vi "filteredWhiteNoise.vi"(9 "frequency":dbl=0.5, 10 "offset":dbl, 11 "amplitude":dbl) -> (2 "Noise":dbl, 3 "Binary Noise":dbl)   [LabVIEW 2020]
uses:
  <vilib>/Simulation/Implementation/Shared/SIMSCR Execution Mode.ctl
  <vilib>/Simulation/Scripting/Companion Diagram/SimConfigNode/SimParams.ctl
  <vilib>/Simulation/Scripting/Companion Diagram/SimConfigNode/_simSolvers.ctl
  <vilib>/Simulation/Param Hierarchy/Typedefs/SIMPH Param Control Actions.ctl
  <vilib>/Simulation/Implementation/Shared/NILVSim_ParamChanged.vi
  <vilib>/Simulation/Implementation/Shared/NILVSim_FinishedLate.vi
  <vilib>/Simulation/Implementation/Shared/NILVSIM_BeginStep.vi
  <vilib>/Simulation/DataSources/Implementation/NILVSim Signal Generator.llb/SIM Signal Generator (scalar).vi
  <vilib>/Simulation/ContinuousLinear/Implementation/NILVSim Transfer Function.llb/SIM Transfer Function Distributor (SISO CD).vi
  <vilib>/Simulation/ContinuousLinear/Implementation/NILVSim Transfer Function.llb/SIM Transfer Function Collector (SISO).vi
  <vilib>/Simulation/Implementation/Shared/SIM Is Init or Final Stage.vi
  <vilib>/Simulation/SignalDisplay/Implementation/NILVSim Time Waveform.llb/SIM Time Waveform (vector).vi
  <vilib>/Simulation/Implementation/Shared/NILVSim_Manager.vi
  <vilib>/Utility/error.llb/Clear Errors.vi
  <vilib>/Simulation/Implementation/Shared/NILVSim_FinalizeModel.vi
  <vilib>/Simulation/Implementation/Shared/SIM Unbundle Sim Info.vi
  <vilib>/Simulation/Implementation/Shared/NILVSim_Initialize.vi
  <vilib>/addons/Control Design/_Model Construction/Special Model Creation.llb/Special Model Creation SubVI/CD Create 1st Order Model.vi
  <vilib>/addons/Control Design/_Frequency Response Analysis/Frequency Response.llb/Frequency Response subVI/cd_Bode (Transfer Function).vi
  <vilib>/addons/Control Design/_Frequency Response Analysis/Frequency Response.llb/Frequency Response subVI/cd_Bandwidth (Transfer Function).vi
  <vilib>/Simulation/Utility/Implementation/NILVSim Get Time and IsAcceptedStep.vi
  <vilib>/Simulation/Implementation/Shared/NILVSim_GetModelError.vi
  <vilib>/Simulation/Implementation/Shared/SIM SimErrorHandler.vi
  <vilib>/Simulation/Implementation/Shared/SIMSH Read Queue.vi
  <vilib>/Simulation/Implementation/Shared/SIM Bundle Sim Info.vi
  <vilib>/Simulation/Scripting/Companion Diagram/SimConfigNode/SimDog.xnode
  <vilib>/Simulation/Implementation/XNodeFramework/SimXNode/SimX.xnode
  <vilib>/addons/Control Design/_Model Construction/NI_CD_Special Model Creation.lvlib
  <vilib>/addons/Control Design/_Model Construction/Model Typedefs.llb/CD General Elements.ctl
  <vilib>/addons/Control Design/_Model Construction/NI_LinSys_Model Typedefs.lvlib
  <vilib>/addons/Control Design/_Model Construction/Model Typedefs.llb/CD Transfer Function Model (SISO).ctl
  <vilib>/addons/Control Design/_Model Construction/Model Typedefs.llb/CD Transfer Function Model (MIMO).ctl
  <vilib>/addons/Control Design/_Frequency Response Analysis/NI_CD_Frequency Response.lvlib
  <vilib>/Simulation/ContinuousLinear/Implementation/NILVSim Transfer Function.llb/SIM Transfer Function (SISO CD).vi
  <vilib>/Simulation/Implementation/Shared/NI_SIM_Implementation.lvlib
panel:
  out "rad/s":dbl
  out "Bode Magnitude":cluster{"W":dbl[], "Magnitude":dbl[]}[](graph)
  out "Bandwidth":dbl=nan format="%.4f"
  out "Filtered Noise Waveform Chart":waveform(dbl)[](graph)
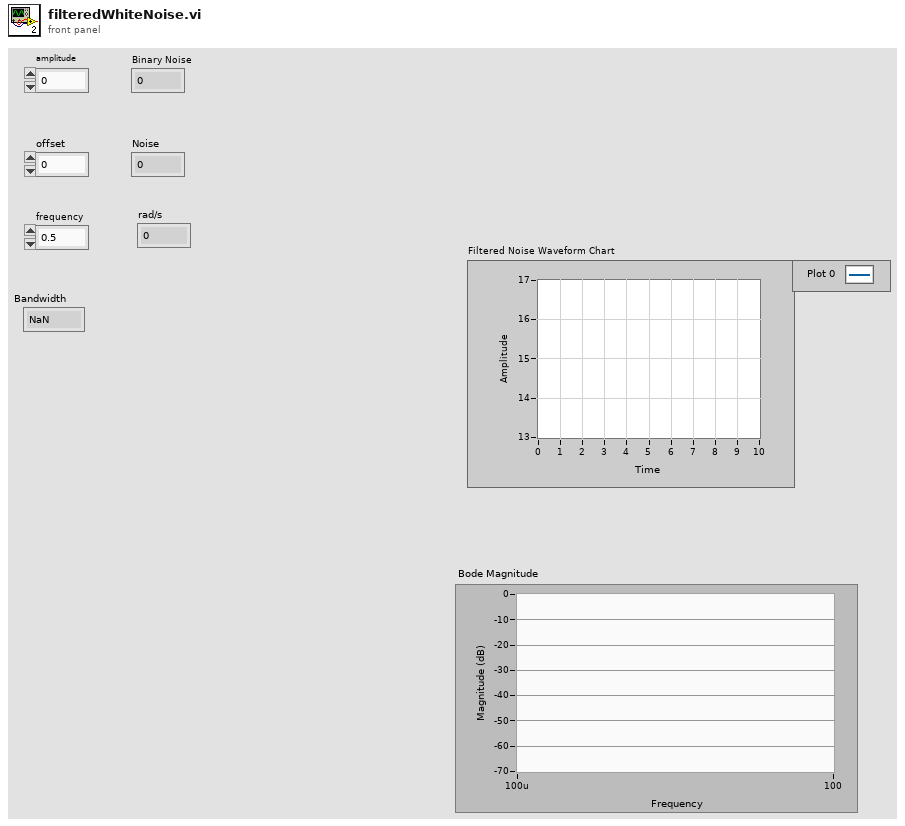
[diagram p1: front panel]
types:
  T1 = typedef "NI_LinSys_Model Typedefs.lvlib/CD Transfer Function Model (MIMO).ctl" = cluster{"properties":T2, "transfer function(s)":T3[][]}
  T2 = typedef "NI_LinSys_Model Typedefs.lvlib/CD General Elements.ctl" = cluster{"Model name":string, "Input names":string[], "Output names":string[], "Input Delays":dbl[], "Output Delays":dbl[], "Sampling Time":dbl, "Notes":string}
  T3 = typedef "NI_LinSys_Model Typedefs.lvlib/CD Transfer Function Model (SISO).ctl" = cluster{"Numerator":dbl[], "Denominator":dbl[], "delay":dbl}
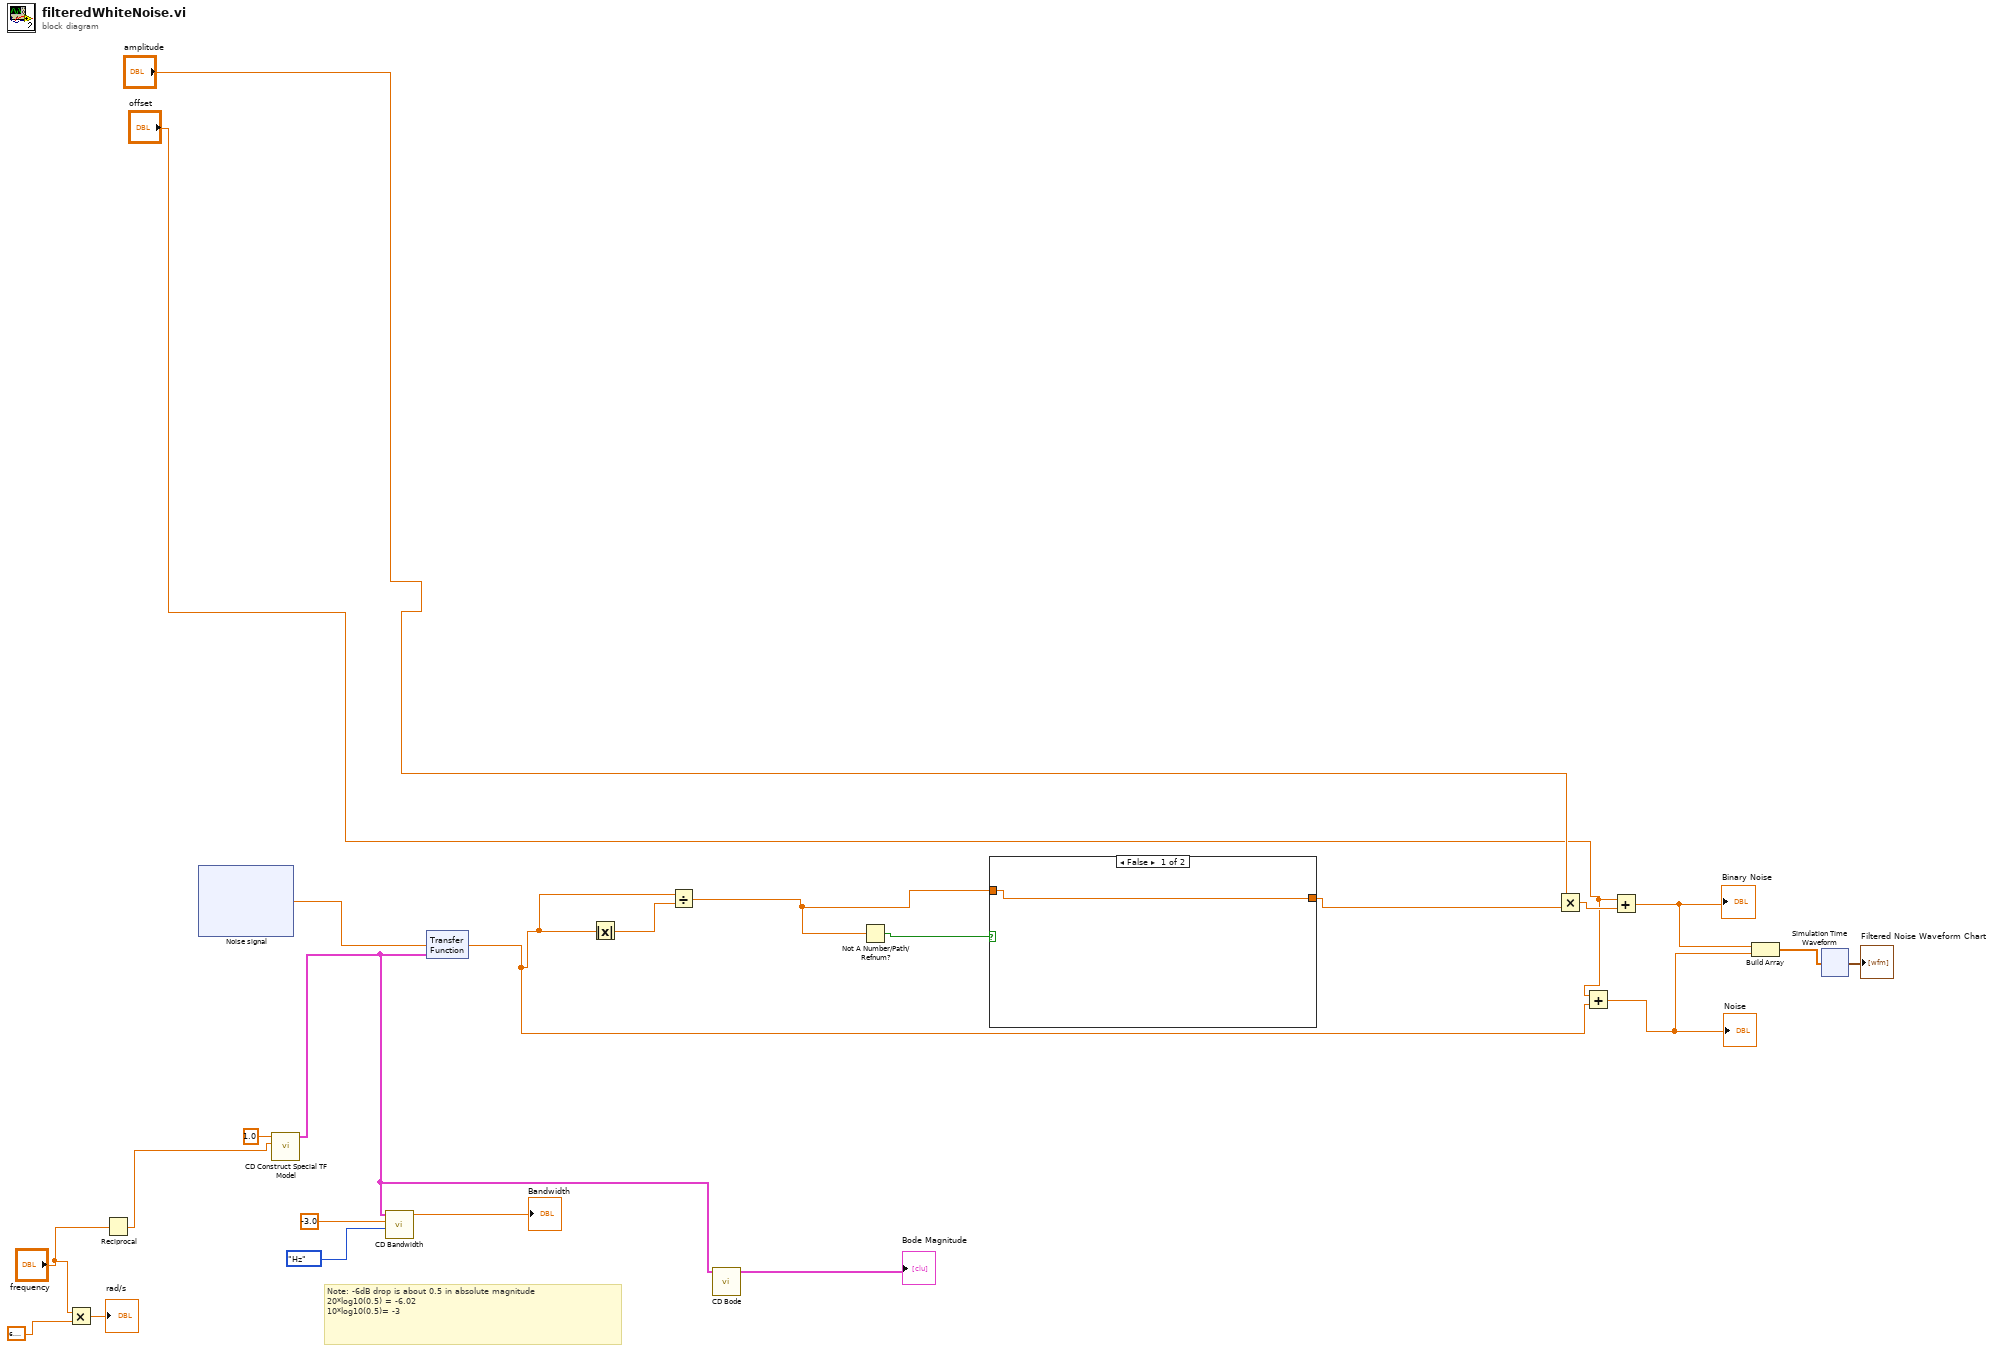
[diagram p0: block diagram]
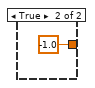
[diagram p2: hidden frame]
diagram:
  # "Note: -6dB drop is about 0.5 in absolute magnitude\n20*log10(0.5) = -6.02\n10*log10(0.5)= -3"
  n1 = Multiply ("Multiply 2")(x="frequency", y=6.283185307179586 ("Constant 2")) -> (x*y=→"rad/s":dbl)
  n2 = Reciprocal(x="frequency") -> (1/x=w17:dbl)
  n3 = xnode "Noise signal"() -> ("output"=w5:dbl)  [unwired: 7 in]
  n4 = call-poly <vilib>:"CD Construct Special TF Model.vi"("Time Constant (s)"=w17, "Static Gain"=1.0) -> ("Transfer Function Model"=w13:T1)  [unwired: 8 in, 1 out]
  n5 = call-poly <vilib>:"CD Bandwidth.vi"("Frequency Unit"=enum16{"Hz", "rad/s"}."Hz", "Magnitude Drop (dB)"=-3.0, "Transfer Function Model"=w13) -> ("Bandwidth"=→"Bandwidth":dbl)  [unwired: 7 in, 1 out]
  n6 = xnode "Transfer Function"("input u(t)"=w5, "Transfer Function"=w13) -> ("output y(t)"=w1:dbl)  [unwired: 2 in, 1 out]
  n7 = Absolute Value(x=w1) -> (abs(x)=w21:dbl)
  n8 = Divide(x=w1, y=w21) -> (x/y=w11:dbl)
  n9 = call-poly <vilib>:"CD Bode.vi"("Transfer Function Model"=w13) -> ("Bode Magnitude"=→"Bode Magnitude":cluster{"W":dbl[], "Magnitude":dbl[]}[])  [unwired: 6 in, 4 out]
  n10 = Not A Number/Path/Refnum?(number/path/refnum=w11) -> (NaN/Path/Refnum?=w12:bool)
  n11 = case shown="False" w12 {
    tunnel: w11 -> [w24 _]
    tunnel: [w24 -1.0 ("Constant")] -> w10
    frame False {
    }
    frame True {
    }
  }
  n12 = Multiply(x="amplitude", y=w10) -> (x*y=w23:dbl)
  n13 = Add ("Add 2")(x="offset", y=w1) -> (x+y=w4:dbl)
  "Noise" <- w4
  n14 = Add(x="offset", y=w23) -> (x+y=w3:dbl)
  "Binary Noise" <- w3
  n15 = Build Array(w3, w4) -> (w2:dbl[])
  n16 = xnode ("Simulation Time Waveform")("Value"=w2) -> ("Waveform Chart"=→"Filtered Noise Waveform Chart":waveform(dbl)[])  [unwired: 1 in]
